vi "v_to_xva.vi"(9 "dt":dbl, 10 "v":dbl) -> (1 "a_out":dbl, 2 "v_out":dbl, 3 "x_out":dbl)   [LabVIEW 2019]
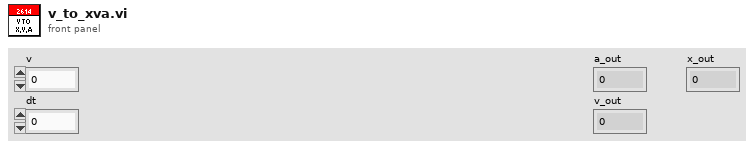
[diagram p1: front panel]
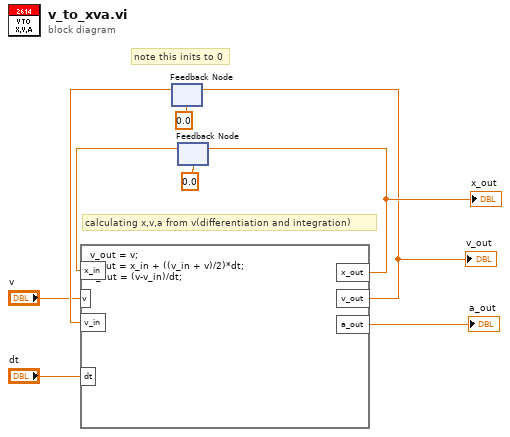
[diagram p0: block diagram]
diagram:
  # "note this inits to 0"
  # "calculating x,v,a from v(differentiation and integration)"
  n1 = feedback #1(0.0 ("input variable")) -> (w4:dbl)
  n2 = feedback #2(0.0 ("input variable")) -> (w6:dbl)
  n3 = formula code="v_out = v;\nx_out = x_in + ((v_in + v)/2)*dt;\na_out = (v-v_in)/dt;"("v_in"=w4, "x_in"=w6, "dt"="dt", "v"="v") -> ("a_out"=→"a_out":dbl, "x_out"=w7:dbl, "v_out"=w5:dbl)
  "v_out" <- w5
  "x_out" <- w7
  n4 = feedback-in #1(w5) -> ()
  n5 = feedback-in #2(w7) -> ()
